vi "port set Name.vi"(6 "bufferLength":i32, 7 "buffer":string, 8 "error in (no error)":errorcluster, 9 "index":i32, 10 "result":cluster{"value":i32, "error":i32}, 11 "id":u32) -> (0 "error out":errorcluster, 2 "result out":cluster{"value":i32, "error":i32}, 3 "id out":u32, 5 "buffer out":string)   [LabVIEW 2014, in "BrainStem2_LabVIEW_Library.lvlib"]
doc: "aLIBEXPORT void __stdcall port_setName ( unsigned int* id, struct Result* result, const int index , unsigned char * buffer, const int bufferLength ) ;"
uses:
  BrainStem2_LabVIEW_Library.lvlib
  BrainStem2_LabVIEW.dll
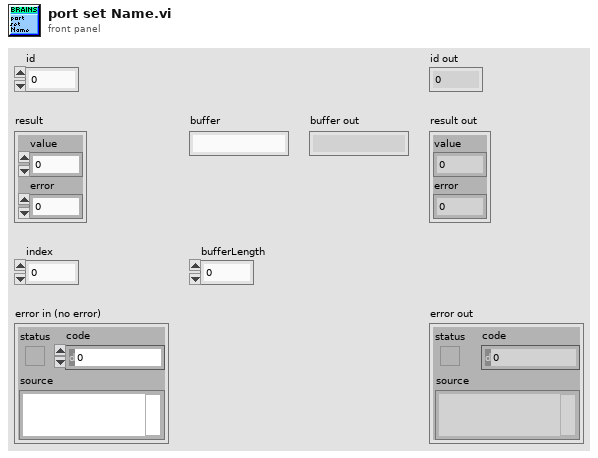
[diagram p1: front panel]
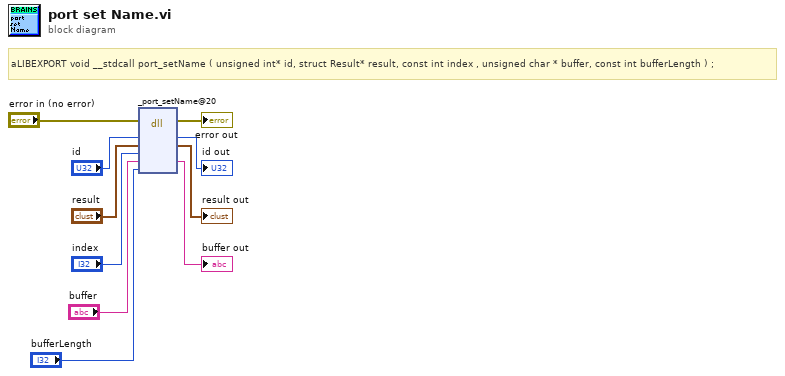
[diagram p0: block diagram]
diagram:
  # "aLIBEXPORT void __stdcall port_setName ( unsigned int* id, struct Result* result, const int index , unsigned char * buffer, const int bufferLength ) ;"
  n1 = dll-call lib="C:/Users/mitch/Documents/development/acroname/software/acroname/aSource/BrainStem2/BrainStem2_LabVIEW/LabVIEW_2014_Distribution/BrainStem2_LabVIEW_w32/BrainStem2_LabVIEW.*" fn="_port_setName@20"(error in="error in (no error)", "id"="id", "result"="result", "index"="index", "buffer"="buffer", "bufferLength"="bufferLength") -> (error out=→"error out":errorcluster, "id"=→"id out":u32, "result"=→"result out":cluster{"value":i32, "error":i32}, "buffer"=→"buffer out":string)  [unwired: 5 in, 1 out]
